vi "SetPDAnotFFT.vi"(1 "set":u8=1, 2 "board_sel":u32=1) -> ()   [LabVIEW 2015]
uses:
  ESLSCDLL.dll
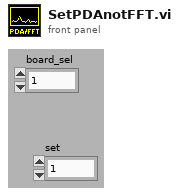
[diagram p1: front panel]
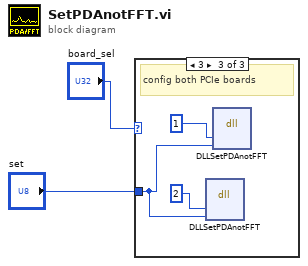
[diagram p0: block diagram]
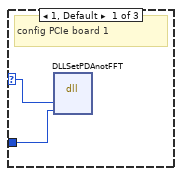
[diagram p2: hidden frame]
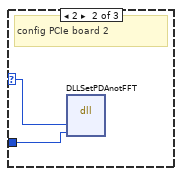
[diagram p3: hidden frame]
diagram:
  n1 = case shown="3" "board_sel" {
    selector: "board_sel" -> [w4 w6 _]
    tunnel: "set" -> [w3 w5 w7]
    frame 1, Default {
      # "config PCIe board 1"
      n2 = dll-call lib="C:/ENTW/PCIE/lv64/board.vis/ESLSCDLL.dll" fn="DLLSetPDAnotFFT" ("lwlscdll.dll:DLLSetISPDA")("drv"=w4, "set"=w3) -> ()  [unwired: 6 in, 2 out]
    }
    frame 2 {
      # "config PCIe board 2"
      n3 = dll-call lib="C:/ENTW/PCIE/lv64/board.vis/ESLSCDLL.dll" fn="DLLSetPDAnotFFT" ("lwlscdll.dll:DLLSetISPDA")("drv"=w6, "set"=w5) -> ()  [unwired: 6 in, 2 out]
    }
    frame 3 {
      # "config both PCIe boards"
      n4 = dll-call lib="C:/ENTW/PCIE/lv64/board.vis/ESLSCDLL.dll" fn="DLLSetPDAnotFFT" ("lwlscdll.dll:DLLSetISPDA")("drv"=u32 2, "set"=w7) -> ()  [unwired: 6 in, 2 out]
      n5 = dll-call lib="C:/ENTW/PCIE/lv64/board.vis/ESLSCDLL.dll" fn="DLLSetPDAnotFFT" ("lwlscdll.dll:DLLSetISPDA")("drv"=u32 1, "set"=w7) -> ()  [unwired: 6 in, 2 out]
    }
  }
